vi "Create_WF_i(t).vi"(8 "error in":errorcluster caption="entrée d'erreur", 10 "N":i32=5, 11 "Position XY (for i(t))":dbl[](array[numeric])=[5.0, 5.0]) -> (0 "error out":errorcluster caption="sortie d'erreur", 2 "Graphe":dbl[][](graph), 3 "Position XY (for i(t)) 2":dbl[][](array[numeric]))   [LabVIEW 2026]
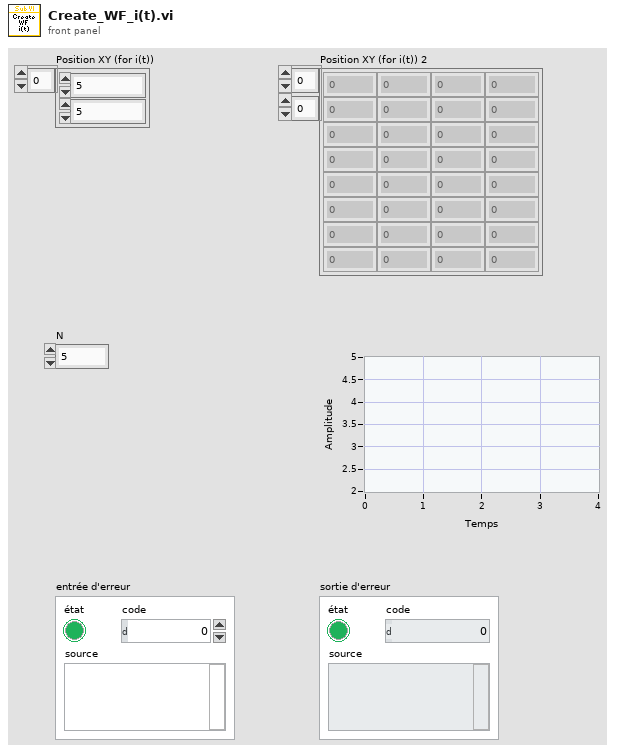
[diagram p1: front panel]
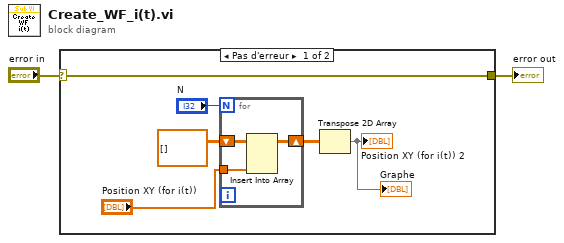
[diagram p0: block diagram]
diagram:
  n1 = case shown="Pas d'erreur" "error in" {
    selector: "error in" -> [w8 w12]
    tunnel: [w8 w12] -> w1
    frame No Error {
      n2 = for {
        N: "N" -> [_]
        tunnel: "Position XY (for i(t))" -> [w10]
        shift-right: [w9] -> w5
        shift-left: dbl[][] [] -> [w11]
        n3 = Insert Into Array(array=w11, new element=w10) -> (w9:dbl[][])  [unwired: 2 in]
      }
      n4 = Transpose 2D Array(2D array=w5) -> (transposed array=→"Position XY (for i(t)) 2" →"Graphe":dbl[][])
    }
    frame Error {
    }
  }
  "error out" <- w1
